vi "Static_Collision.vi"() -> ()   [LabVIEW 2010]
uses:
  Facet_Array.ctl
panel:
  in  "Dynamic Facets":T1
  in  "Static Facets":T1
  in  "Read Files":path
  in  "Body Centroid":dbl[](array[numeric])
  in  "Body Bubble Rad":dbl
  in  "No of Dynamic Facets":i32
  in  "No of Static Facets":i32
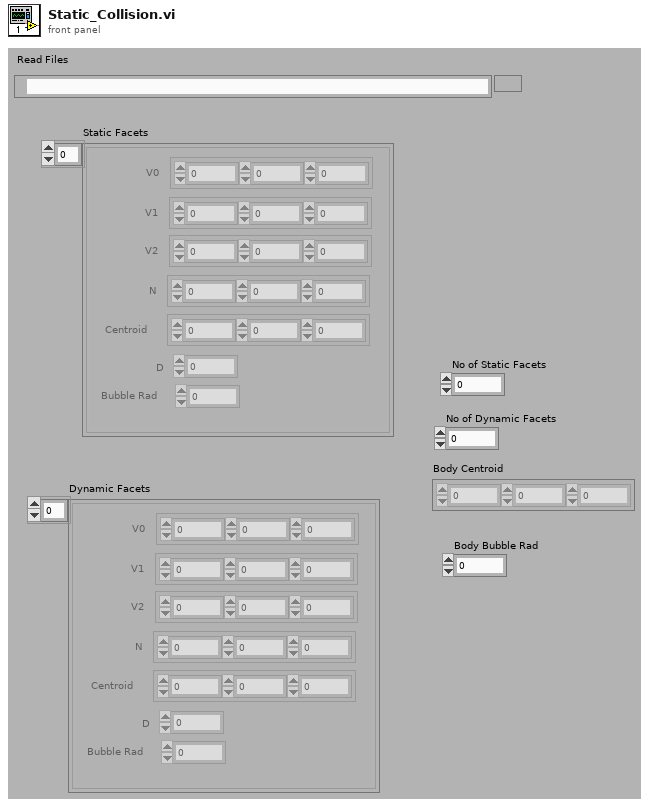
[diagram p1: front panel]
types:
  T1 = typedef "Facet_Array.ctl" = cluster{"V0":dbl[], "V1":dbl[], "V2":dbl[], "N":dbl[], "Centroid":dbl[], "D":dbl, "Bubble Rad":dbl}[]
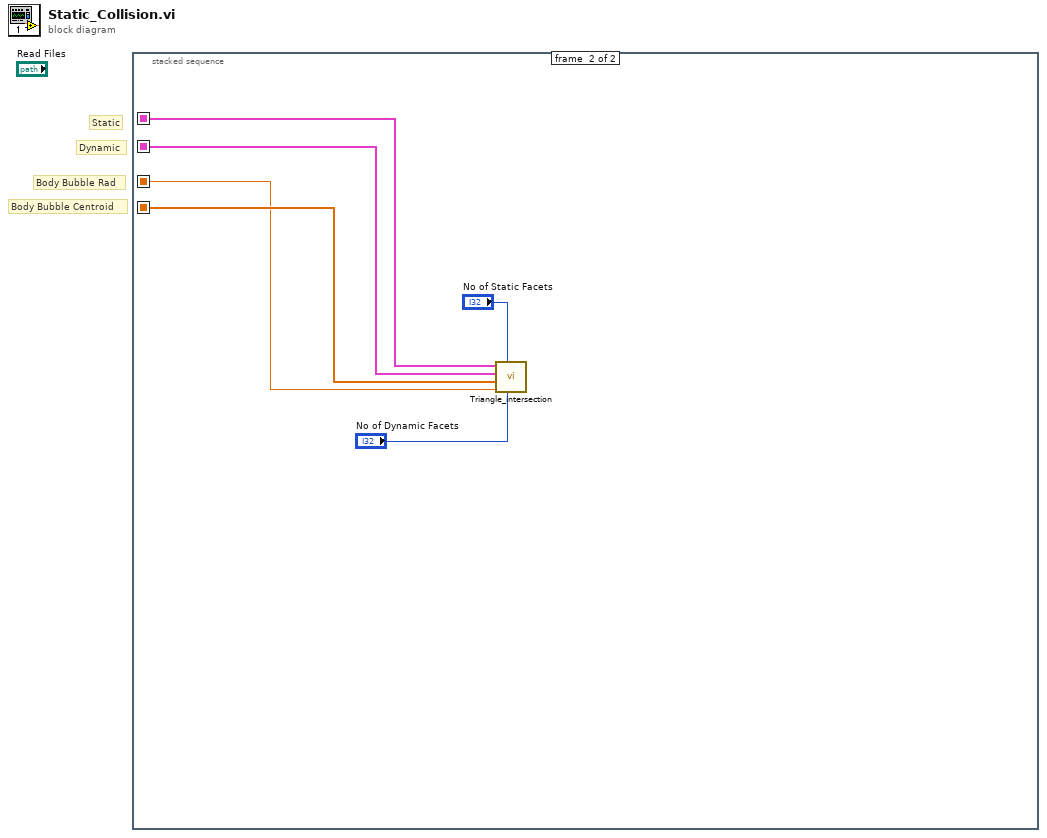
[diagram p0: block diagram]
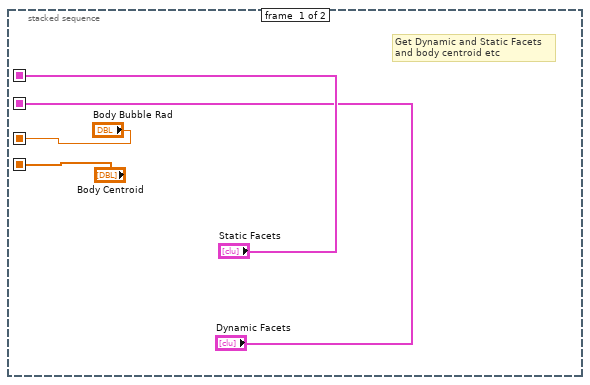
[diagram p2: hidden frame]
diagram:
  # "Body Bubble Centroid"
  # "Body Bubble Rad"
  # "Dynamic"
  # "Static"
  n1 = stacked-sequence {
    seq-local: ["Static Facets" _] -> [_ w10]
    seq-local: ["Dynamic Facets" _] -> [_ w9]
    seq-local: ["Body Bubble Rad" _] -> [_ w7]
    seq-local: ["Body Centroid" _] -> [_ w8]
    frame #0 {
      # "Get Dynamic and Static Facets\nand body centroid etc"
    }
    frame #1 {
      n2 = call "Triangle_intersection.vi"("No of Dynamic Facets"="No of Dynamic Facets", "No of Static Facets"="No of Static Facets", "Body Bubble Rad"=w7, "Body Centroid"=w8, "Dynamic Facets"=w9, "Static Facets"=w10) -> ()  [unwired: 1 out]
    }
  }
